vi "LVClass_WavefrontCorrector Check Actuator User Preferences.vi"(0 "WavefrontCorrector in":refnum<class "WavefrontCorrector.lvclass">, 5 "Index of actuator":i32, 7 "Wavefront Corrector State":T1, 11 "error in (no error)":errorcluster) -> (4 "WavefrontCorrector out":refnum<class "WavefrontCorrector.lvclass">, 15 "error out":errorcluster)   [LabVIEW 2020, in "WavefrontCorrector.lvclass"]
doc: "Assert requested preferences fulfill specifications constraints.\n\n<B>correctorIn</B> : WavefrontCorrector object.\n<B>correctorOut</B> : WavefrontCorrector object.\n<B>actuator_index</B> : Index of the actuator.\n<B>min</B> : WavefrontCorrector actuator preferences : lowest command value.\n<B>max</B> : WavefrontCorrector actuator preferences : highest command value.\n<B>validity</B> : WavefrontCorrector actuator preferences : status.\n<B>fixed_value</B> : WavefrontCorrector actuator preferences : fixed positions."
uses:
  WavefrontCorrector.lvclass
  Controls/Wavefront Corrector states - ONE.ctl
  WavefrontCorrector.lvclass/WavefrontCorrector.ctl
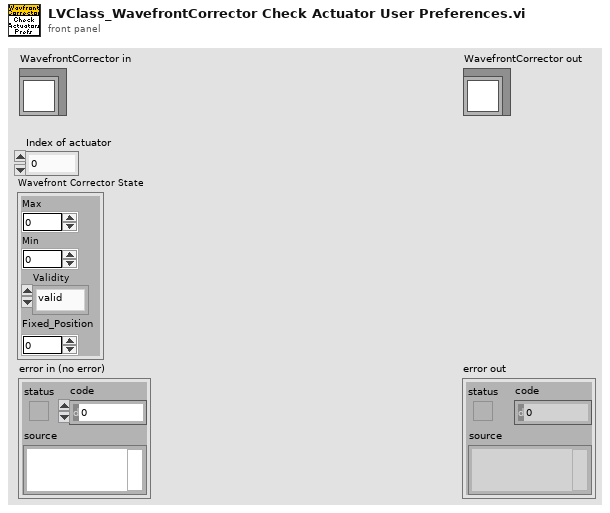
[diagram p1: front panel]
types:
  T1 = typedef "Wavefront Corrector states - ONE.ctl" = cluster{"Max":sgl, "Min":sgl, "Validity":enum16{"valid", "fixed", "invalid"}, "Fixed_Position":sgl}
  T2 = typedef "ClassID.ctl" = i64
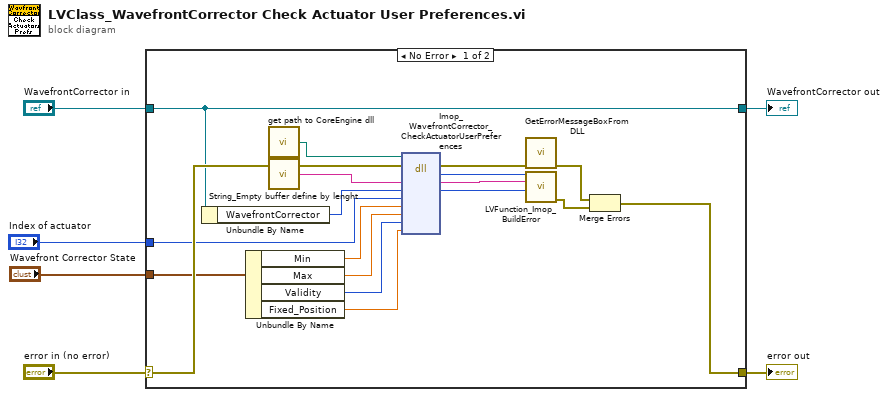
[diagram p0: block diagram]
diagram:
  n1 = case shown="No Error" "error in (no error)" {
    selector: "error in (no error)" -> [w17 w26]
    tunnel: [w16 w26] -> w5
    tunnel: [w14 w25] -> w3
    tunnel: "WavefrontCorrector in" -> [w14 w25]
    tunnel: "Wavefront Corrector State" -> [w15 _]
    tunnel: "Index of actuator" -> [w12 _]
    frame No Error {
      n2 = Unbundle By Name(w14) -> ("WavefrontCorrector"=w13:T2)
      n3 = Unbundle By Name(w15) -> ("Min"=w11:sgl, "Max"=w10:sgl, "Validity"=w9:enum16{"valid", "fixed", "invalid"}, "Fixed_Position"=w8:sgl)
      n4 = call "get path to CoreEngine dll.vi"() -> ("path to wavekit library"=w24:path)  [unwired: 14 in, 1 out]
      n5 = call "String_Empty buffer define by lenght.vi"() -> ("Empty buffer"=w23:string)  [unwired: 1 in]
      n6 = dll-call lib="D:/FLE/0.Code/CoreEngine4_Suite/LV2011_interface/DLLs/c_interface_vc100.dll" fn="Imop_WavefrontCorrector_CheckActuatorUserPreferences"(path in=w24, error in=w17, "Message"=w23, "WavefrontCorrector"=w13, "Index of actuator"=w12, "Min"=w11, "Max"=w10, "Validity"=w9, "Fixed position"=w8) -> (error out=w22:errorcluster, "return type"=w20:i32, "Message"=w21:string, "WavefrontCorrector"=w7:i64)  [unwired: 6 in, 1 out]
      n7 = call "GetErrorMessageBoxFromDLL.vi"("error IN"=w22) -> ("error OUT"=w18:errorcluster)  [unwired: 10 in]
      n8 = call "LVFunction_Imop_BuildError.vi"("code"=w20, "String to Prepend to source (\"\")"=w21, "Adresse"=w7) -> ("error out"=w19:errorcluster)  [unwired: 12 in]
      n9 = Merge Errors(w18, w19) -> (w16:errorcluster)
    }
    frame Error {
    }
  }
  "error out" <- w5
  "WavefrontCorrector out" <- w3
